vi "Look for Cold.vi"   [LabVIEW 2013]
uses:
  Robot Global Data.vi
  <vilib>/Rock Robotics/WPI/RobotDrive/WPI_RobotDriveMecanumDrive_Cartesian.vi
  <vilib>/Rock Robotics/WPI/RobotDrive/WPI_RobotDriveGetSetRefNum.vi
types:
  T1 = typedef "WPI_RobotDriveDevRef.ctl" = cluster{"DevStatus":errorcluster, "Motors[]":T2[], "Square Inputs":bool, "Max Output":dbl, "Isochronous":bool}
  T2 = typedef "WPI_MotorControlDeviceRef.ctl" = cluster{"DeviceStatus":errorcluster, "Type":enum16{"PWM", "CAN"}, "PWM":cluster{"Digital Module":T3, "PWM Channel":T4, "DeadBand":T5}, "CAN":cluster{"Device Number":u8, "Control Mode":T6, "Semaphore":T7, "Max Vout":dbl}, "Invert":bool, "TransformRef":T8, "InvTransformRef":T8}
  T3 = typedef "FPGA_TypedefDigitalModule.ctl" = enum16{"Digital Module 1", "Digital Module 2"}
  T4 = typedef "FPGA_DIOPWMChannel.ctl" = enum8{"PWM 1", "PWM 2", "PWM 3", "PWM 4", "PWM 5", "PWM 6", "PWM 7", "PWM 8", "PWM 9", "PWM 10", "Invalid"}
  T5 = typedef "WPI_PWMDeadband.ctl" = cluster{"Name":string, "maxPositivePwm":i32, "minPositivePwm":i32, "centerPwm":i32, "maxNegativePwm":i32, "minNegativePwm":i32, "angularRange":u16}
  T6 = typedef "WPI_CANJaguar_ControlMode.ctl" = enum8{"Percent VBus", "Current", "Speed", "Position", "Voltage"}
  T7 = typedef "Semaphore RefNum" = refnum<k1>
  T8 = typedef "WPI_PWMTransform_ConPane.ctl" = refnum<vi>
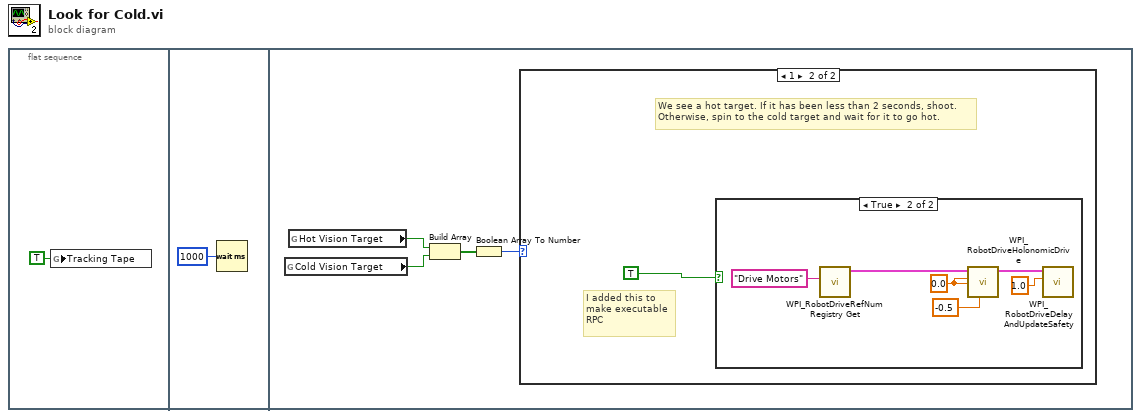
[diagram p0: block diagram]
diagram:
  n1 = flat-sequence {
    frame #0 {
      n2 = global write "Robot Global Data.vi" "Tracking Tape"(TRUE ("Enable Vision")) -> ()
    }
    frame #1 {
      n3 = Wait (ms)(milliseconds to wait=u32 1000) -> ()  [unwired: 1 out]
    }
    frame #2 {
      n4 = global read "Robot Global Data.vi" "Cold Vision Target"() -> (w6:bool)
      n5 = global read "Robot Global Data.vi" "Hot Vision Target"() -> (w5:bool)
      n6 = Build Array(w5, w6) -> (w4:bool[])
      n7 = Boolean Array To Number(Boolean array=w4) -> (number=w3:u32)
      n8 = case shown="1" w3 {
        frame 0, Default {
        }
        frame 1 {
          # "I added this to\nmake executable\nRPC"
          # "We see a hot target. If it has been less than 2 seconds, shoot.\nOtherwise, spin to the cold target and wait for it to go hot."
          n9 = case shown="True" TRUE {
            frame False {
            }
            frame True {
              w9 = 0.0 ("Rotation")
              n10 = call <vilib>:"WPI_RobotDriveRefNum Registry Get.vi"("refnum name"="Drive Motors") -> ("RobotDriveDevRef"=w13:T1)  [unwired: 1 in, 9 out]
              n11 = call-poly <vilib>:"WPI_RobotDriveHolonomicDrive.vi"("Rotation"=-0.5, "Y"=w9, "X"=w9, "RobotDriveDevRef"=w13) -> ("RobotDriveDevRef"=w10:T1)  [unwired: 5 in, 2 out]
              n12 = call <vilib>:"WPI_RobotDriveDelayAndUpdateSafety.vi"("Delay (s)"=1.0, "RobotDriveDevRef"=w10) -> ()  [unwired: 8 in, 2 out]
            }
          }
        }
      }
    }
  }
